vi "Camera Stream Video Writer.vi"() -> ()   [LabVIEW 2014]
doc: "A more complex demonstration is the use of a camera stream in comination with a video writer.\nThe grabbed images from the stream are written to a file on the disk.\n\nWhen you succesfully wrote a file, you can check the demo \"File Stream\" to read it."
uses:
  MSC Image_class/MSC Image.lvclass
  MSC Video_class/MSC Video.lvclass
  MSC Video Writer_class/MSC Video Writer.lvclass
panel:
  in  "CamID":i32
  in  "Path":path=path "Browse for Path ->"
  in  "FPS":u32=30
  out "error out":errorcluster
  in  "stop":bool
  out "Live Image":picture
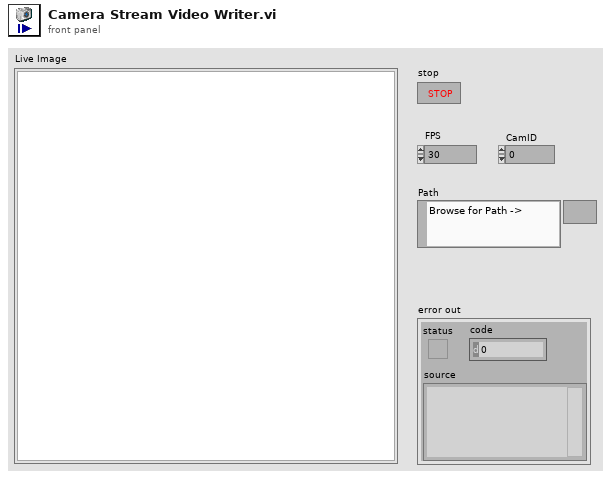
[diagram p1: front panel]
types:
  T1 = typedef "MSC Image.lvclass/Size.ctl" = cluster{"Cols":i32, "Rows":i32}
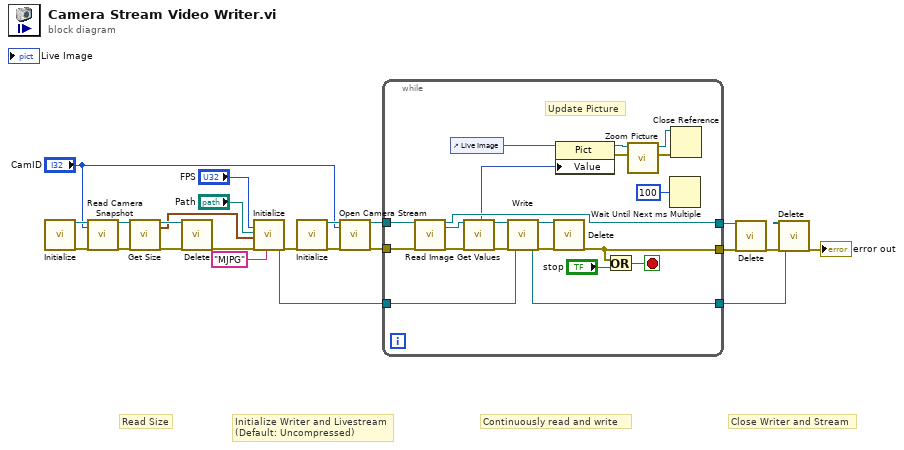
[diagram p0: block diagram]
diagram:
  # "Close Writer and Stream"
  # "Continuously read and write"
  # "Initialize Writer and Livestream\n(Default: Uncompressed)"
  # "Read Size"
  n1 = call "Initialize.vi"() -> ("image out"=w10:refnum<class "MSC Image.lvclass">, "error out"=w7:errorcluster)  [unwired: 18 in]
  n2 = call-dynamic "Read Camera Snapshot.vi"("image in"=w10, "camID"="CamID", "error in (no error)"=w7) -> ("image out"=w9:refnum<class "MSC Image.lvclass">, "error out"=w6:errorcluster)  [unwired: 15 in]
  n3 = call-dynamic "Get Size.vi"("image in"=w9, "error in (no error)"=w6) -> ("image out"=w8:refnum<class "MSC Image.lvclass">, "Size"=w4:T1, "error out"=w5:errorcluster)  [unwired: 15 in]
  n4 = call-dynamic "Delete.vi"("image in"=w8, "error in (no error)"=w5) -> ("error out"=w2:errorcluster)  [unwired: 17 in]
  n5 = call "Initialize.vi"("FPS"="FPS", "Path"="Path", "Size"=w4, "error in (no error)"=w2, "FourCC Codec"="MJPG") -> ("video writer out"=w18:refnum<class "MSC Video Writer.lvclass">, "error out"=w14:errorcluster)  [unwired: 13 in]
  n6 = call "Initialize.vi"("error in (no error)"=w14) -> ("video out"=w23:refnum<class "MSC Video.lvclass">, "error out"=w13:errorcluster)  [unwired: 17 in]
  n7 = call-dynamic "Open Camera Stream.vi"("video in"=w23, "CamID"="CamID", "error in (no error)"=w13) -> ("video out"=w22:refnum<class "MSC Video.lvclass">, "error out"=w21:errorcluster)  [unwired: 15 in]
  n8 = while {
    tunnel: w22 -> [w44]
    tunnel: w21 -> [w43]
    tunnel: [w41] -> w20
    tunnel: [w38] -> w19
    tunnel: w18 -> [w29]
    tunnel: [w26] -> w17
    stop <- w42 stop-if-true
    # "Update Picture"
    n9 = call-dynamic "Read Image.vi"("video in"=w44, "error in (no error)"=w43) -> ("video out"=w41:refnum<class "MSC Video.lvclass">, "image out"=w25:refnum<class "MSC Image.lvclass">, "error out"=w40:errorcluster)  [unwired: 15 in]
    n10 = control-ref of="Live Image"() -> (w37:refnum<vi>)
    n11 = call-dynamic "Get Values.vi"("image in"=w25, "error in (no error)"=w40) -> ("picture"=w32:picture, "image out"=w31:refnum<class "MSC Image.lvclass">, "error out"=w28:errorcluster)  [unwired: 10 in, 5 out]
    n12 = call-dynamic "Write.vi"("video writer in"=w29, "image in"=w31, "error in (no error)"=w28) -> ("video writer out"=w26:refnum<class "MSC Video Writer.lvclass">, "image out"=w30:refnum<class "MSC Image.lvclass">, "error out"=w27:errorcluster)  [unwired: 14 in]
    n13 = call-dynamic "Delete.vi"("image in"=w30, "error in (no error)"=w27) -> ("error out"=w38:errorcluster)  [unwired: 17 in]
    n14 = property class="Pict"(reference=w37, "Value"=w32) -> (reference out=w33:refnum<vi>, error out=w34:errorcluster)  [unwired: 1 in]
    n15 = Or(x=w38, y="stop") -> (x .or. y?=w42:bool)
    n16 = call "Zoom Picture.vi"("error in (no error)"=w34, "Picture in"=w33) -> ("error out"=w36:errorcluster, "Picture out"=w35:refnum<vi>)  [unwired: 8 in]
    n17 = Wait Until Next ms Multiple(millisecond multiple=u32 100) -> ()  [unwired: 1 out]
    n18 = Close Reference(reference=w35, error in (no error)=w36) -> ()  [unwired: 1 out]
  }
  n19 = call-dynamic "Delete.vi"("video in"=w20, "error in (no error)"=w19) -> ("error out"=w16:errorcluster)  [unwired: 17 in]
  n20 = call-dynamic "Delete.vi"("video writer in"=w17, "error in (no error)"=w16) -> ("error out"=→"error out":errorcluster)  [unwired: 17 in]
